vi "OpenG Array filter - Scalar Regexp Template.vi"() -> ()   [LabVIEW 2012]
panel:
  out "filtered item indices":i32[](array[numeric])
  out "filtered array":string[](array[string])
  in  "items to filter":string
  in  "Array Input":string[](array[string])
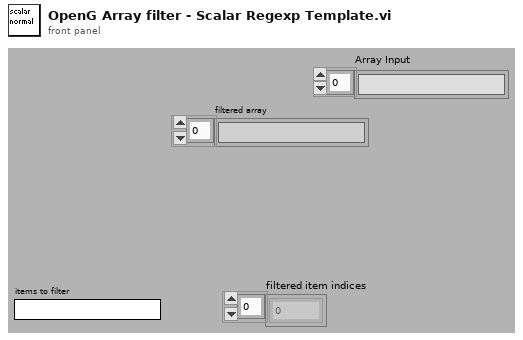
[diagram p1: front panel]
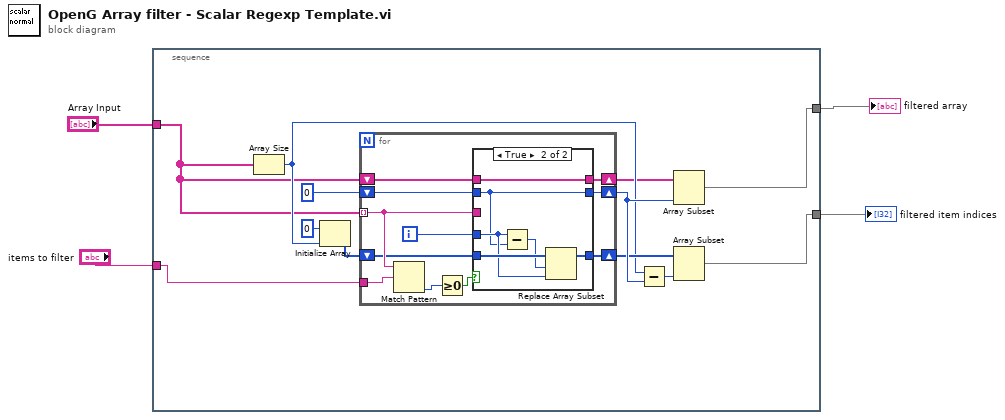
[diagram p0: block diagram]
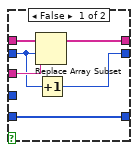
[diagram p2: hidden frame]
diagram:
  n1 = stacked-sequence {
    tunnel: "items to filter" -> [w8]
    tunnel: [w6] -> w3
    tunnel: "Array Input" -> [w7]
    tunnel: [w5] -> w1
    frame #0 {
      n2 = Array Size(array=w7) -> (size(s)=w13:i32)
      n3 = Initialize Array(0 ("Numeric"), w13) -> (w12:i32[])
      n4 = for {
        tunnel: w7 -> [w25] mode=indexing
        shift-right: [w26] -> w10
        shift-left: w7 -> [w27]
        shift-right: [w23] -> w15
        shift-left: 0 -> [w24]
        shift-right: [w21] -> w14
        shift-left: w12 -> [w22]
        tunnel: w8 -> [w20]
        i -> [w19]
        n5 = Match Pattern(string=w25, regular expression=w20) -> (offset past match=w18:i32)  [unwired: 4 out]
        n6 = Greater Or Equal To 0?(x=w18) -> (x >= 0?=w17:bool)
        n7 = case shown="True" w17 {
          tunnel: w27 -> [w33 w39]
          tunnel: [w32 w39] -> w26
          tunnel: w25 -> [w31 _]
          tunnel: w24 -> [w29 w35]
          tunnel: [w30 w35] -> w23
          tunnel: w22 -> [w28 w38]
          tunnel: [w28 w37] -> w21
          tunnel: w19 -> [_ w36]
          frame False {
            n8 = Replace Array Subset(array=w33, new element=w31, index=w29) -> (w32:string[])
            n9 = Increment(x=w29) -> (x+1=w30:i32)
          }
          frame True {
            n10 = Subtract(x=w36, y=w35) -> (x-y=w34:i32)
            n11 = Replace Array Subset(array=w38, new element=w36, index=w34) -> (w37:i32[])
          }
        }
      }
      n12 = Subtract(x=w13, y=w15) -> (x-y=w16:i32)
      n13 = Array Subset(array=w10, length=w15) -> (w5:string[])  [unwired: 1 in]
      n14 = Array Subset(array=w14, length=w16) -> (w6:i32[])  [unwired: 1 in]
    }
  }
  "filtered array" <- w1
  "filtered item indices" <- w3
